vi "Xcor1D (SubVI).vi"(5 "corner-based Coordinates (pix)":dbl[](array[numeric]), 6 "Original Data":i16[][](array[numeric]), 7 "stripe halfwidth":i8=9) -> (2 "corner-based coordinates":dbl[](array[numeric]), 3 "center-based coordinates":dbl[](array[numeric]))   [LabVIEW 2011, in "OfflineTracker.lvlib"]
uses:
  OfflineTracker.lvlib
  <vilib>/Analysis/NI_AALBase.lvlib
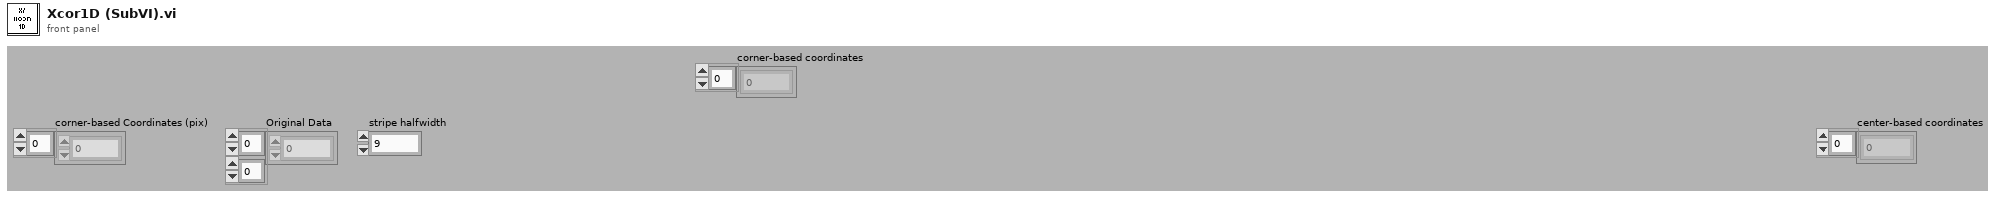
[diagram p1: front panel]
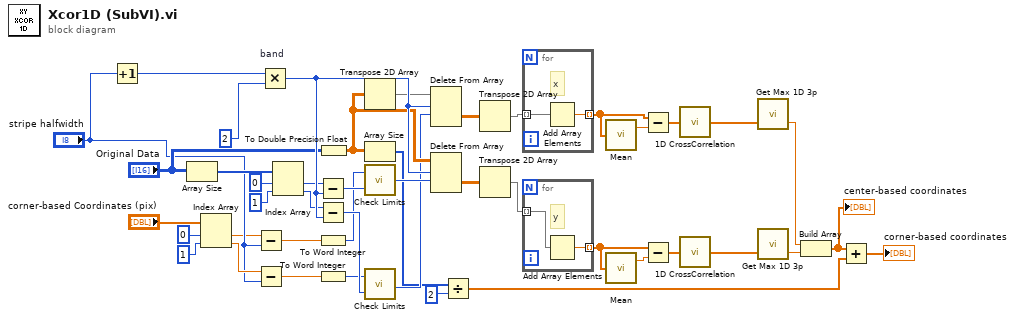
[diagram p0: block diagram]
diagram:
  n1 = Increment(x="stripe halfwidth") -> (x+1=w31:i8)
  n2 = Array Size(array="Original Data") -> (size(s)=w36:i32[])
  n3 = Index Array(array="corner-based Coordinates (pix)", index #1=0 ("index"), index #2=1 ("index")) -> (element #1=w18:dbl, element #2=w38:dbl)
  n4 = Subtract(x=w18, y="stripe halfwidth") -> (x-y=w19:dbl)
  n5 = Subtract(x=w38, y="stripe halfwidth") -> (x-y=w20:dbl)
  n6 = Multiply "band"(x=w31, y=i8 2) -> (x*y=w44:i8)
  n7 = Index Array(array=w36, index #1=0 ("index"), index #2=1 ("index")) -> (element #1=w43:i32, element #2=w41:i32)
  n8 = Subtract(x=w43, y=w44) -> (x-y=w42:i32)
  n9 = Subtract(x=w41, y=w44) -> (x-y=w40:i32)
  n10 = To Word Integer(number=w19) -> (16bit integer=w25:i16)
  n11 = To Word Integer(number=w20) -> (16bit integer=w22:i16)
  n12 = To Double Precision Float(number="Original Data") -> (double precision float=w32:dbl[][])
  n13 = Transpose 2D Array(2D array=w32) -> (transposed array=w5:dbl[][])
  n14 = Array Size(array=w32) -> (size(s)=w1:i32[])
  n15 = call "Check Limits.vi"("Max Value"=w42, "Input"=w25) -> ("Output"=w24:i16)
  n16 = call "Check Limits.vi"("Max Value"=w40, "Input"=w22) -> ("Output"=w23:i16)
  n17 = Delete From Array(array=w5, length=w44, index (row)=w23) -> (deleted portion=w9:dbl[][])  [unwired: 1 in, 1 out]
  n18 = Delete From Array(array=w32, length=w44, index (row)=w24) -> (deleted portion=w7:dbl[][])  [unwired: 1 in, 1 out]
  n19 = Divide(x=w1, y=2) -> (x/y=w2:dbl[])
  n20 = Transpose 2D Array(2D array=w9) -> (transposed array=w21:dbl[][])
  n21 = Transpose 2D Array(2D array=w7) -> (transposed array=w8:dbl[][])
  n22 = for {
    tunnel: w21 -> [w46] mode=indexing
    tunnel: [w45] -> w15 mode=indexing
    # "x"
    n23 = Add Array Elements(numeric array=w46) -> (sum=w45:dbl)
  }
  n24 = for {
    tunnel: w8 -> [w48] mode=indexing
    tunnel: [w47] -> w12 mode=indexing
    # "y"
    n25 = Add Array Elements(numeric array=w48) -> (sum=w47:dbl)
  }
  n26 = call <vilib>:"Mean.vi"("X"=w15) -> ("mean"=w16:dbl)  [unwired: 1 out]
  n27 = call <vilib>:"Mean.vi"("X"=w12) -> ("mean"=w13:dbl)  [unwired: 1 out]
  n28 = Subtract(x=w15, y=w16) -> (x-y=w14:dbl[])
  n29 = Subtract(x=w12, y=w13) -> (x-y=w11:dbl[])
  n30 = call "1D CrossCorrelation.vi"("Intensity Profile"=w14) -> ("CrossCorrelation"=w6:dbl[])
  n31 = call "1D CrossCorrelation.vi"("Intensity Profile"=w11) -> ("CrossCorrelation"=w10:dbl[])
  n32 = call "Get Max 1D 3p.vi"("CrossCorrelation"=w6) -> ("Position"=w28:dbl)  [unwired: 1 in, 1 out]
  n33 = call "Get Max 1D 3p.vi"("CrossCorrelation"=w10) -> ("Position"=w27:dbl)  [unwired: 1 in, 1 out]
  n34 = Build Array(w28, w27) -> (w4:dbl[])
  "center-based coordinates" <- w4
  n35 = Add(x=w4, y=w2) -> (x+y=→"corner-based coordinates":dbl[])
